vi "Global 6.vi"() -> ()   [LabVIEW 2019]
panel:
  in  "Numeric":i32
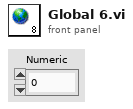
[diagram p1: front panel]
diagram:
